vi "TXT Report_Init.vi"(8 "error in (no error)":errorcluster) -> (0 "error out":errorcluster, 3 "TXT_Report out":refnum<class "TXT Report.lvclass">)   [LabVIEW 2009, in "TXT Report.lvclass"]
doc: "This VI defines the object type for a TXT Report.\n\nAAL 9/09"
uses:
  TXT Report.lvclass
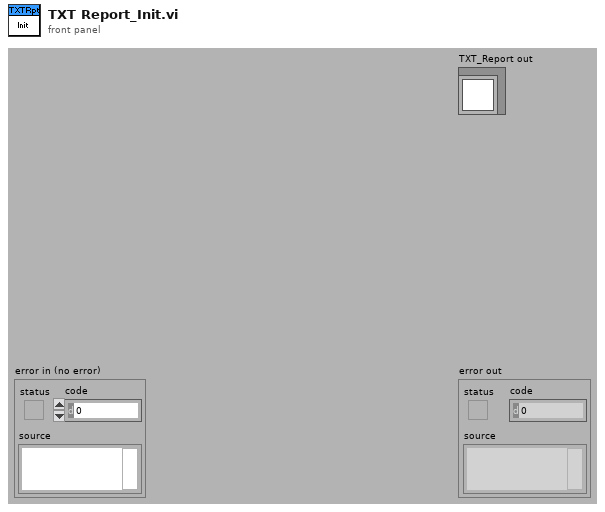
[diagram p1: front panel]
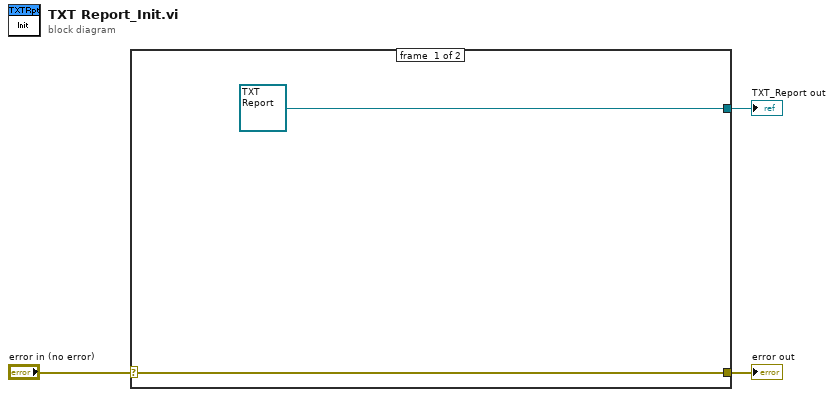
[diagram p0: block diagram]
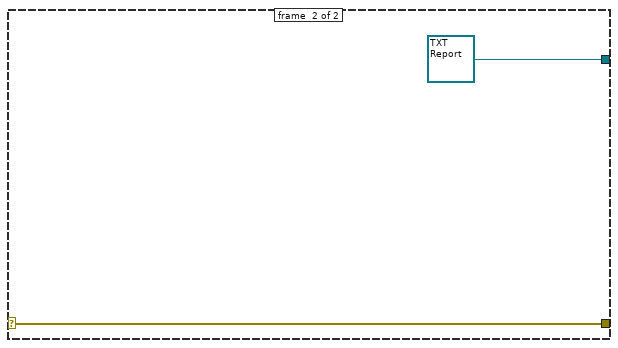
[diagram p2: hidden frame]
diagram:
  n1 = case shown="No Error" "error in (no error)" {
    selector: "error in (no error)" -> [w4 w7]
    tunnel: [w4 w7] -> w2
    tunnel: [refnum<class "TXT Report.lvclass"> refnum ("TXT_Report.lvclass") refnum<class "TXT Report.lvclass"> refnum ("TXT_Report.lvclass")] -> w1
    frame #0 {
    }
    frame #1 {
    }
  }
  "error out" <- w2
  "TXT_Report out" <- w1
